vi "Distance Between Two Points.vi"(10 "Point 2":T1 {"Latitude" format="%#_10g"; "Longitude" format="%#_10g"}, 11 "Point 1":T1 {"Latitude" format="%#_10g"; "Longitude" format="%#_10g"}) -> (3 "Distance (km)":dbl)   [LabVIEW 2014]
uses:
  Controls/PointLatLon.ctl
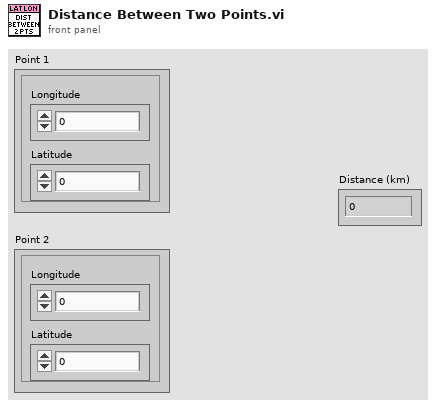
[diagram p1: front panel]
types:
  T1 = typedef "PointLatLon.ctl" = cluster{"Longitude":dbl, "Latitude":dbl}
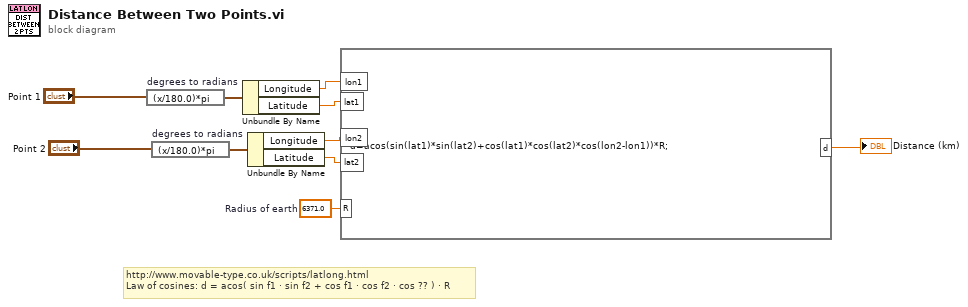
[diagram p0: block diagram]
diagram:
  w9 = 6371.0  # Radius of earth
  # "http://www.movable-type.co.uk/scripts/latlong.html\nLaw of cosines:\td = acos( sin f1 · sin f2 + cos f1 · cos f2 · cos ?? ) · R"
  n1 = expression code="(x/180.0)*pi" "degrees to radians"("Point 1") -> (w10:T1)
  n2 = expression code="(x/180.0)*pi" "degrees to radians"("Point 2") -> (w3:T1)
  n3 = Unbundle By Name(w10) -> ("Longitude"=w7:dbl, "Latitude"=w6:dbl)
  n4 = Unbundle By Name(w3) -> ("Longitude"=w2:dbl, "Latitude"=w1:dbl)
  n5 = formula code="d=acos(sin(lat1)*sin(lat2)+cos(lat1)*cos(lat2)*cos(lon2-lon1))*R;"("lon1"=w7, "lat1"=w6, "R"=w9, "lon2"=w2, "lat2"=w1) -> ("d"=→"Distance (km)":dbl)
